vi "korona2012.vi"() -> ()   [LabVIEW 2010]
panel:
  in  "record":bool
  in  "clear":bool
  in  "proc":bool
  in  "stop":bool
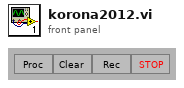
[diagram p1: front panel]
types:
  T1 = enum16{"Left Button", "Center Button", "Right Button", "Window Close"}
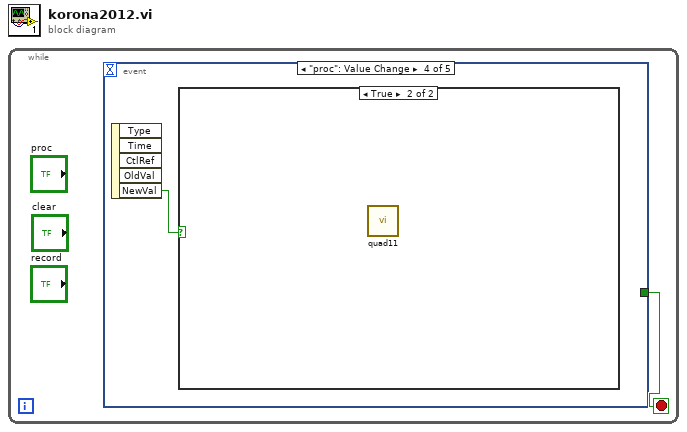
[diagram p0: block diagram]
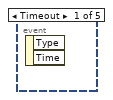
[diagram p2: hidden frame]
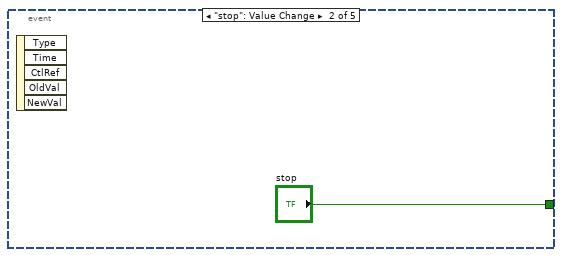
[diagram p3: hidden frame]
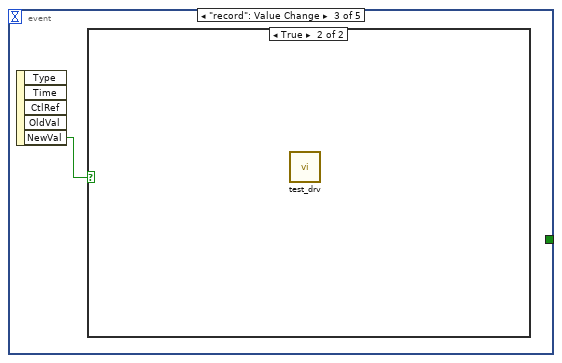
[diagram p4: hidden frame]
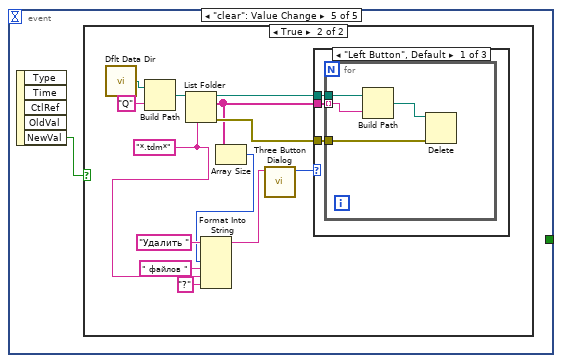
[diagram p7: hidden frame]
diagram:
  n1 = while {
    stop <- w1 stop-if-true
    n2 = event shown="[3] \"proc\": Value Change" {
      selector: _ -> [_ _ _ _ _]
      dyn-events: _ -> [_ _ _ _ _]
      timeout: _ -> [_ _ _ _ _]
      tunnel: [_ "stop" _ _ _] -> w1
      event Timeout {
        n3 = event-data() -> ()  [unwired: 1 in, 2 out]
      }
      event "stop": Value Change {
        n4 = event-data() -> ()  [unwired: 1 in, 5 out]
      }
      event "record": Value Change {
        n5 = event-data() -> ("NewVal"=w3:bool)  [unwired: 1 in, 4 out]
        n6 = case shown="True" w3 {
          frame False {
          }
          frame True {
            n7 = call "test_drv.vi"() -> ()  [unwired: 1 in]
          }
        }
      }
      event "proc": Value Change {
        n8 = event-data() -> ("NewVal"=w4:bool)  [unwired: 1 in, 4 out]
        n9 = case shown="True" w4 {
          frame False {
          }
          frame True {
            n10 = call "quad11.vi"() -> ()  [unwired: 12 in]
          }
        }
      }
      event "clear": Value Change {
        n11 = event-data() -> ("NewVal"=w5:bool)  [unwired: 1 in, 4 out]
        n12 = case shown="True" w5 {
          frame False {
          }
          frame True {
            w9 = "*.tdm*" ("pattern")
            n13 = call <vilib>:"Dflt Data Dir.vi"() -> ("App:Default Data Directory"=w18:path)
            n14 = Build Path(base path=w18, name or relative path="Q") -> (appended path=w16:path)
            n15 = List Folder(path=w16, pattern=w9) -> (path out=w15:path, filenames=w11:string[], error out=w14:errorcluster)  [unwired: 2 in, 1 out]
            n16 = Array Size(array=w11) -> (size(s)=w10:i32)
            n17 = Format Into String(initial string="Удалить ", w10, " файлов " ("input 2"), w9, "?" ("input 4")) -> (resulting string=w6:string)  [unwired: 2 in, 1 out]
            n18 = call <vilib>:"Three Button Dialog.vi"("message"=w6) -> ("Which Button?"=w13:T1)  [unwired: 10 in]
            n19 = case shown="\"Left Button\", Default" w13 {
              tunnel: w11 -> [w21 _ _]
              tunnel: w15 -> [w20 _ _]
              tunnel: w14 -> [w19 _ _]
              frame "Left Button", Default {
                n20 = for {
                  tunnel: w21 -> [w24] mode=indexing
                  tunnel: w20 -> [w25]
                  tunnel: w19 -> [w22]
                  n21 = Build Path(base path=w25, name or relative path=w24) -> (appended path=w23:path)
                  n22 = Delete(path (use dialog)=w23, error in=w22) -> ()  [unwired: 3 in, 3 out]
                }
              }
              frame "Center Button" {
              }
              frame "Right Button" {
              }
            }
          }
        }
      }
    }
  }
